vi "Gunsim Vision Adapter.vi"(1 "Other Constants":T1={"Ball Diameter(in)"=10.0, "Air Density(g/in^3)"=0.02, "Drag coefficient"=0.5, "Ball Mass(g)"=300.0, "gravity(in/s^2)"=-386.09, "Minimum Goal Height(in)"=90.0, "Maximum Goal Height(in)"=104.0}, 2 "Horizontal Distance":dbl[](array[numeric])) -> (0 "cluster out":T2)   [LabVIEW 2015]
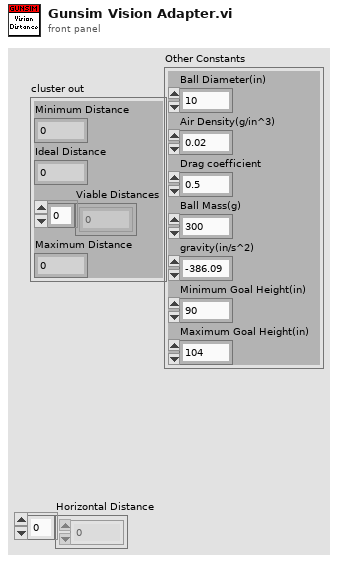
[diagram p1: front panel]
types:
  T1 = cluster{"Ball Diameter(in)":dbl, "Air Density(g/in^3)":dbl, "Drag coefficient":dbl, "Ball Mass(g)":dbl, "gravity(in/s^2)":dbl, "Minimum Goal Height(in)":dbl, "Maximum Goal Height(in)":dbl}
  T2 = cluster{"Minimum Distance":dbl, "Ideal Distance":dbl, "Viable Distances":dbl[], "Maximum Distance":dbl}
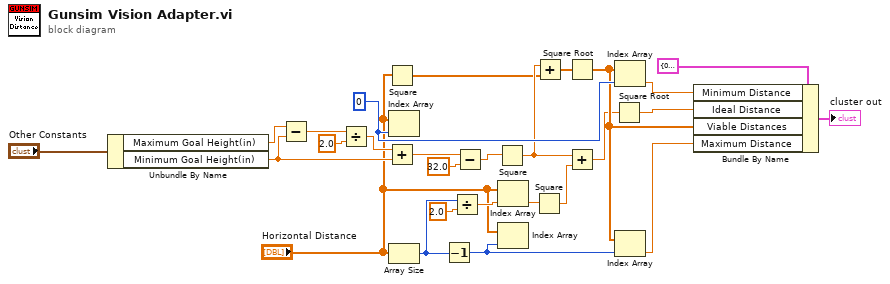
[diagram p0: block diagram]
diagram:
  w21 = 0 ("index")
  n1 = Unbundle By Name("Other Constants") -> ("Maximum Goal Height(in)"=w9:dbl, "Minimum Goal Height(in)"=w5:dbl)
  n2 = Subtract(x=w9, y=w5) -> (x-y=w7:dbl)
  n3 = Divide(x=w7, y=2.0) -> (x/y=w6:dbl)
  n4 = Square(x="Horizontal Distance") -> (x^2=w17:dbl[])
  n5 = Add(x=w6, y=w5) -> (x+y=w2:dbl)
  n6 = Index Array(array="Horizontal Distance", index=w21) -> ()  [unwired: 1 out]
  n7 = Array Size(array="Horizontal Distance") -> (size(s)=w25:i32)
  n8 = Decrement(x=w25) -> (x-1=w22:i32)
  n9 = Divide(x=w25, y=2.0) -> (x/y=w24:dbl)
  n10 = Subtract(x=w2, y=32.0) -> (x-y=w1:dbl)
  n11 = Square(x=w1) -> (x^2=w18:dbl)
  n12 = Index Array(array="Horizontal Distance", index=w24) -> (element=w26:dbl)
  n13 = Index Array(array="Horizontal Distance", index=w22) -> ()  [unwired: 1 out]
  n14 = Square(x=w26) -> (x^2=w15:dbl)
  n15 = Add(x=w18, y=w17) -> (x+y=w16:dbl[])
  n16 = Square Root(x=w16) -> (sqrt(x)=w19:dbl[])
  n17 = Add(x=w18, y=w15) -> (x+y=w14:dbl)
  n18 = Square Root(x=w14) -> (sqrt(x)=w27:dbl)
  n19 = Index Array(array=w19, index=w21) -> (element=w12:dbl)
  n20 = Index Array(array=w19, index=w22) -> (element=w13:dbl)
  n21 = Bundle By Name(cluster=T2 {"Minimum Distance"=0.0, "Ideal Distance"=0.0, "Viable Distances"=[], "Maximum Distance"=0.0} ("input cluster"), "Minimum Distance"=w12, "Ideal Distance"=w27, "Viable Distances"=w19, "Maximum Distance"=w13) -> (→"cluster out":T2)
